vi "Test_Email.vi"() -> ()   [LabVIEW 2010]
uses:
  Controls/Post_Process.ctl
  Globals/Meas_global.vi
panel:
  in  "error in (no error)":errorcluster={"status"=TRUE, "code"=0, "source"="hello"}
  out "Continue":bool
  out "SMS Message":string
  out "Email Message":string
  in  "Error Type":string="Paul_test"
  in  "Dialog Box (T)":bool
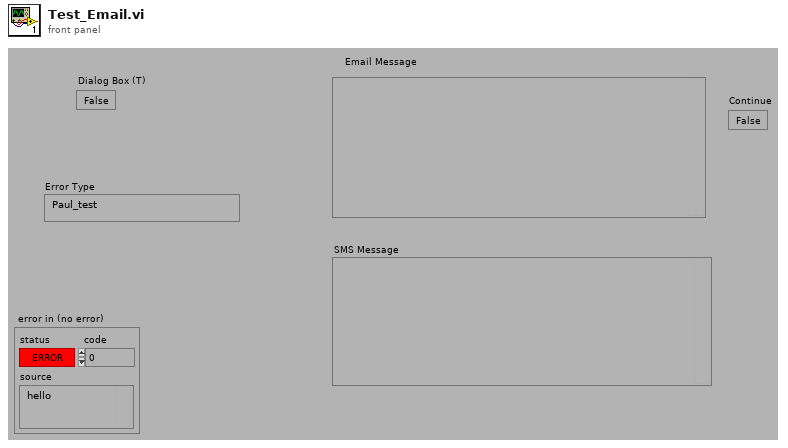
[diagram p1: front panel]
types:
  T1 = typedef "Post_Process.ctl" = enum16{"Take New Data", "Post Process Raw Data File"}
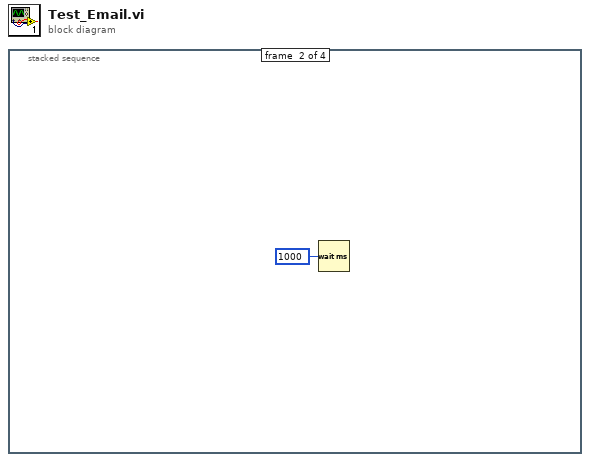
[diagram p0: block diagram]
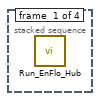
[diagram p2: hidden frame]
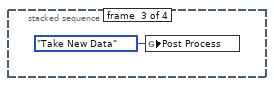
[diagram p3: hidden frame]
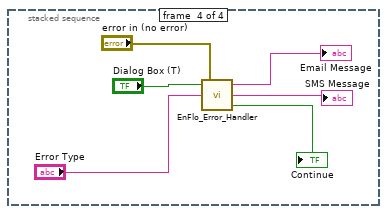
[diagram p4: hidden frame]
diagram:
  n1 = stacked-sequence {
    frame #0 {
      n2 = call "Run_EnFlo_Hub.vi"() -> ()  [unwired: 8 in]
    }
    frame #1 {
      n3 = Wait (ms)(milliseconds to wait=u32 1000) -> ()  [unwired: 1 out]
    }
    frame #2 {
      n4 = global write "Meas_global.vi" "Post Process"(Post_Process."Take New Data" ("Post Process")) -> ()
    }
    frame #3 {
      n5 = call "EnFlo_Error_Handler.vi"("error in (no error)"="error in (no error)", "Error Type"="Error Type", "Dialog Box (T)"="Dialog Box (T)") -> ("Continue"=→"Continue":bool, "SMS Message"=→"SMS Message":string, "Email Message"=→"Email Message":string)
    }
  }
